vi "Get Active Cell Index.vi"(8 "error in (no error)":errorcluster, 11 "DataGridView in":refnum<class "DataGridView.lvclass">) -> (0 "error out":errorcluster, 1 "ColumnIndex":i32, 2 "RowIndex":i32, 3 "DataGridView out":refnum<class "DataGridView.lvclass">)   [LabVIEW 2013, in "DataGrid.lvlib" / "DataGridView.lvclass"]
uses:
  DataGridView.lvclass
  DataGridView.lvclass/DataGridView.ctl
  System.Windows.Forms
  Properties/Read DataGridView.vi
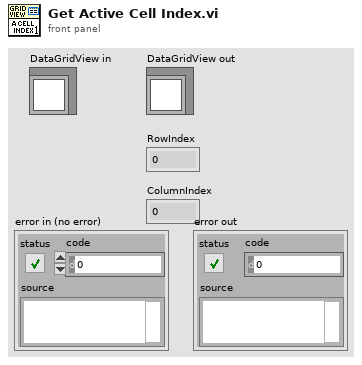
[diagram p1: front panel]
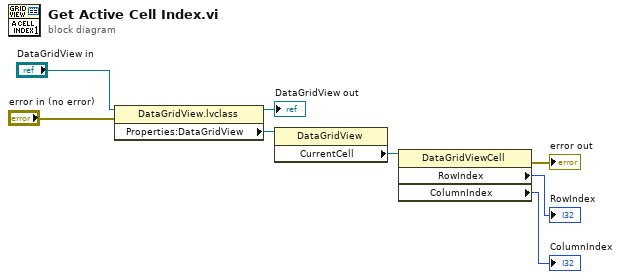
[diagram p0: block diagram]
diagram:
  n1 = property class="DataGridView.lvclass"(reference="DataGridView in", error in="error in (no error)") -> (reference out=→"DataGridView out":refnum<class "DataGridView.lvclass">, "Properties:DataGridView"=w5:refnum<k24>)  [unwired: 1 out]
  n2 = property class="DataGridView"(reference=w5) -> ("CurrentCell"=w6:refnum<k24>)  [unwired: 1 in, 2 out]
  n3 = property class="DataGridViewCell"(reference=w6) -> (error out=→"error out":errorcluster, "RowIndex"=→"RowIndex":i32, "ColumnIndex"=→"ColumnIndex":i32)  [unwired: 1 in, 1 out]
